vi "ScaleXCoordinate.vi"(1 "Scale":dbl=-1.0 format="%#_13g", 2 "X, Y, Z Input":dbl[](array[numeric]) format="%#_13g") -> (0 "c * X, Y, Z Output":dbl[](array[numeric]))   [LabVIEW 2016]
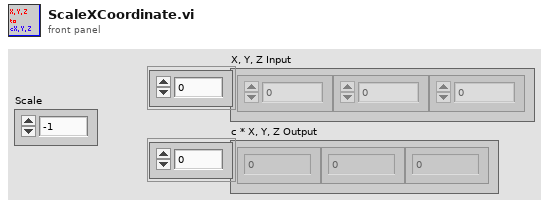
[diagram p1: front panel]
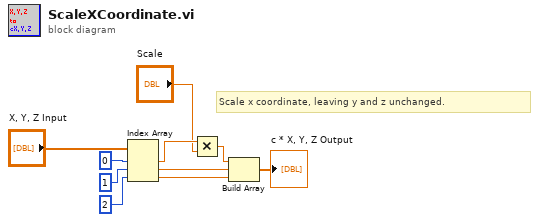
[diagram p0: block diagram]
diagram:
  # "Scale x coordinate, leaving y and z unchanged."
  n1 = Index Array(array="X, Y, Z Input", index #1=0 ("index"), index #2=1 ("index"), index #3=2 ("index")) -> (element #1=w6:dbl, element #2=w3:dbl, element #3=w2:dbl)
  n2 = Multiply(x=w6, y="Scale") -> (x*y=w4:dbl)
  n3 = Build Array(w4, w3, w2) -> (→"c * X, Y, Z Output":dbl[])
